vi "LED Strip.vi"   [LabVIEW 2013]
uses:
  <vilib>/Rock Robotics/WPI/Solenoid/WPI_SolenoidValue.ctl
  <vilib>/Rock Robotics/WPI/Solenoid/WPI_SolenoidSetEnum.vi
types:
  T1 = typedef "WPI_DriverStationAllianceInfo.ctl" = enum16{"Red", "Blue", "Invalid"}
  T2 = typedef "WPI_SolenoidValue.ctl" = enum16{"Off", "On", "Forward", "Reverse"}
  T3 = typedef "WPI_SolenoidDevRef.ctl" = cluster{"DevStatus":errorcluster, "Solenoid Module":T4, "Forward Solenoid Channel":T5, "Reverse Solenoid Channel":T5}
  T4 = typedef "FPGA_TypedefSolenoidModule.ctl" = enum16{"Solenoid Module 1", "Solenoid Module 2"}
  T5 = typedef "WPI_SolenoidChannel.ctl" = enum8{"Solenoid 1", "Solenoid 2", "Solenoid 3", "Solenoid 4", "Solenoid 5", "Solenoid 6", "Solenoid 7", "Solenoid 8", "Invalid"}
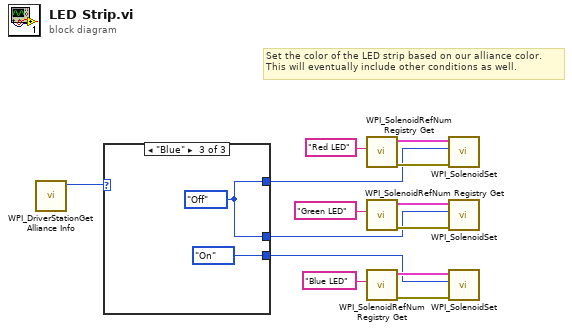
[diagram p0: block diagram]
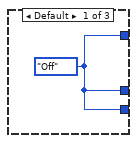
[diagram p2: hidden frame]
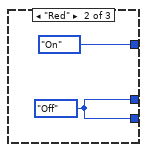
[diagram p3: hidden frame]
diagram:
  # "Set the color of the LED strip based on our alliance color.\nThis will eventually include other conditions as well."
  n1 = call <vilib>:"WPI_DriverStationGet Alliance Info.vi"() -> ("Alliance"=w11:T1)  [unwired: 10 in, 1 out]
  n2 = case shown="\"Blue\"" w11 {
    tunnel: [w14 WPI_SolenoidValue."On" ("Value") w17] -> w3
    tunnel: [w14 w16 w17] -> w2
    tunnel: [w14 w16 WPI_SolenoidValue."On" ("Value")] -> w1
    frame Default {
      w14 = WPI_SolenoidValue."Off" ("Value")
    }
    frame "Red" {
      w16 = WPI_SolenoidValue."Off" ("Value")
    }
    frame "Blue" {
      w17 = WPI_SolenoidValue."Off" ("Value")
    }
  }
  n3 = call <vilib>:"WPI_SolenoidRefNum Registry Get.vi"("refnum name"="Red LED") -> ("error out"=w13:errorcluster, "SolenoidDevRef"=w12:T3)  [unwired: 9 in]
  n4 = call <vilib>:"WPI_SolenoidRefNum Registry Get.vi"("refnum name"="Green LED") -> ("error out"=w9:errorcluster, "SolenoidDevRef"=w8:T3)  [unwired: 9 in]
  n5 = call <vilib>:"WPI_SolenoidRefNum Registry Get.vi"("refnum name"="Blue LED") -> ("error out"=w6:errorcluster, "SolenoidDevRef"=w5:T3)  [unwired: 9 in]
  n6 = call-poly <vilib>:"WPI_SolenoidSet.vi"("error in (no error)"=w13, "Value"=w3, "SolenoidDevRef"=w12) -> ()  [unwired: 7 in, 2 out]
  n7 = call-poly <vilib>:"WPI_SolenoidSet.vi"("error in (no error)"=w9, "Value"=w2, "SolenoidDevRef"=w8) -> ()  [unwired: 7 in, 2 out]
  n8 = call-poly <vilib>:"WPI_SolenoidSet.vi"("error in (no error)"=w6, "Value"=w1, "SolenoidDevRef"=w5) -> ()  [unwired: 7 in, 2 out]
